vi "calculateAbsAmount.vi"() -> ()   [LabVIEW 2023]
panel:
  out "output":dbl
  in  "input":csg
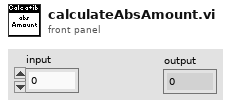
[diagram p1: front panel]
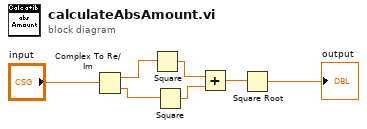
[diagram p0: block diagram]
diagram:
  n1 = Complex To Re/Im(x + iy="input") -> (x=w6:sgl, y=w5:sgl)
  n2 = Square(x=w6) -> (x^2=w4:sgl)
  n3 = Square(x=w5) -> (x^2=w3:sgl)
  n4 = Add(x=w4, y=w3) -> (x+y=w2:sgl)
  n5 = Square Root(x=w2) -> (sqrt(x)=→"output":sgl)
